vi "createCameraLog.vi"(8 "error in (no error)":errorcluster, 11 "CameraController in":refnum<class "CameraController.lvclass">) -> (0 "error out":errorcluster, 2 "Log out":refnum<class "Log.lvclass">, 3 "CameraController out":refnum<class "CameraController.lvclass">)   [LabVIEW 2009, in "Hardware.lvlib" / "Channels.lvlib" / "CameraController.lvclass"]
uses:
  CameraController.lvclass
  Tools/Log.lvclass
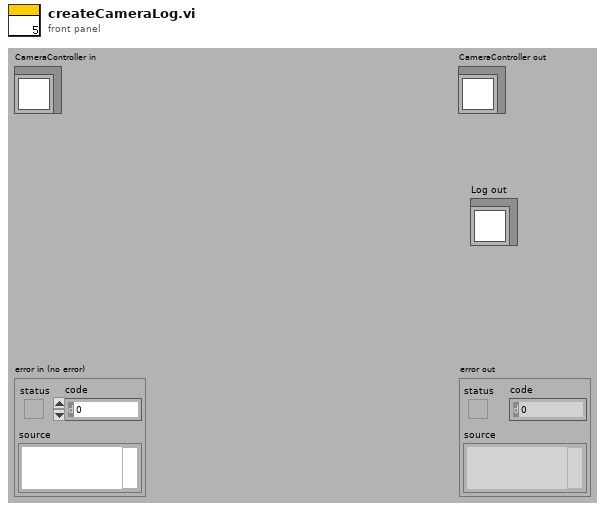
[diagram p1: front panel]
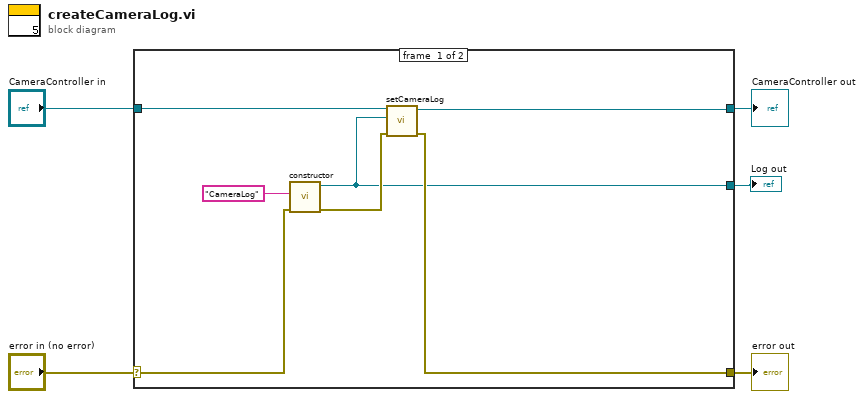
[diagram p0: block diagram]
diagram:
  n1 = case shown="No Error" "error in (no error)" {
    selector: "error in (no error)" -> [w12 w14]
    tunnel: [w7 w14] -> w4
    tunnel: [w8 w13] -> w2
    tunnel: "CameraController in" -> [w10 w13]
    tunnel: [w6 _] -> w1
    frame #0 {
      n2 = call "constructor.vi"("error in (no error)"=w12, "Log Title"="CameraLog") -> ("error out"=w9:errorcluster, "Log out"=w6:refnum<class "Log.lvclass">)  [unwired: 8 in]
      n3 = call-dynamic "setCameraLog.vi"("error in (no error)"=w9, "Tools.lvlib:Log.lvclass"=w6, "CameraController.lvclass in"=w10) -> ("error out"=w7:errorcluster, "CameraController.lvclass out"=w8:refnum<class "CameraController.lvclass">)  [unwired: 7 in]
    }
    frame #1 {
    }
  }
  "error out" <- w4
  "CameraController out" <- w2
  "Log out" <- w1
